vi "IncludeProject.vi"(8 "error in (no error)":errorcluster, 10 "Path":path, 11 "Whitelist in":refnum<class "Whitelist.lvclass">) -> (0 "error out":errorcluster, 3 "Whitelist out":refnum<class "Whitelist.lvclass">)   [LabVIEW 2019, in "Whitelist.lvclass"]
doc: "Includes files from a project in the whitelist."
uses:
  Whitelist.lvclass
  Whitelist.lvclass/Whitelist.ctl
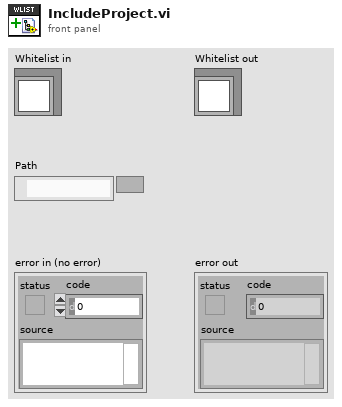
[diagram p1: front panel]
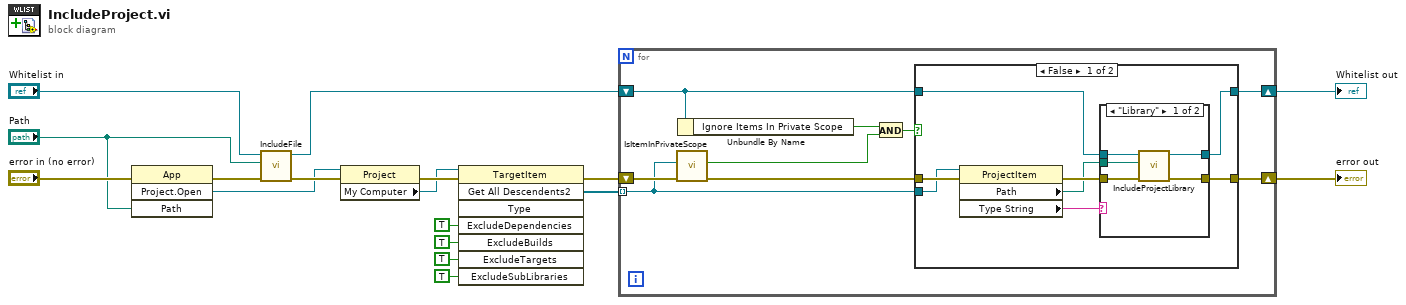
[diagram p0: block diagram]
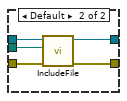
[diagram p2: hidden frame]
diagram:
  n1 = invoke class="App" method="Project.Open"(error in="error in (no error)", "Path"="Path") -> (error out=w16:errorcluster, "Project:Open"=w10:refnum<vi>)  [unwired: 2 in, 2 out]
  n2 = call "IncludeFile.vi"("error in (no error)"=w16, "Path"="Path", "Whitelist in"="Whitelist in") -> ("error out"=w15:errorcluster, "Whitelist out"=w4:refnum<class "Whitelist.lvclass">)  [unwired: 7 in]
  n3 = property class="Project"(reference=w10, error in=w15) -> (error out=w11:errorcluster, "My Computer"=w9:refnum<vi>)  [unwired: 1 out]
  n4 = invoke class="TargetItem" method="Get All Descendents2"(reference=w9, error in=w11, "ExcludeDependencies"=TRUE, "ExcludeBuilds"=TRUE, "ExcludeTargets"=TRUE, "ExcludeSubLibraries"=TRUE) -> (error out=w12:errorcluster, "Get All Descendents2"=w2:refnum<vi>[])  [unwired: 2 in, 6 out]
  n5 = for {
    shift-right: [w26] -> w5
    shift-left: w12 -> [w24]
    shift-right: [w25] -> w3
    shift-left: w4 -> [w20]
    tunnel: w2 -> [w22] mode=indexing
    n6 = call "IsItemInPrivateScope.vi"("error in (no error)"=w24, "Item"=w22) -> ("error out"=w23:errorcluster, "Is Private?"=w19:bool)  [unwired: 8 in]
    n7 = Unbundle By Name(w20) -> ("Ignore Items In Private Scope"=w21:bool)
    n8 = And(x=w21, y=w19) -> (x .and. y?=w18:bool)
    n9 = case shown="False" w18 {
      tunnel: [w34 w45] -> w26
      tunnel: [w33 w46] -> w25
      tunnel: w23 -> [w30 w45]
      tunnel: w22 -> [w29 _]
      tunnel: w20 -> [w28 w46]
      frame False {
        n10 = property class="ProjectItem"(reference=w29, error in=w30) -> (error out=w32:errorcluster, "Path"=w31:path, "Type String"=w27:string)  [unwired: 1 out]
        n11 = case shown="\"Library\"" w27 {
          tunnel: [w38 w44] -> w34
          tunnel: [w35 w43] -> w33
          tunnel: w32 -> [w39 w42]
          tunnel: w31 -> [w36 w41]
          tunnel: w28 -> [w37 w40]
          frame "Library" {
            n12 = call "IncludeProjectLibrary.vi"("error in (no error)"=w39, "Path"=w36, "Whitelist in"=w37) -> ("error out"=w38:errorcluster, "Whitelist out"=w35:refnum<class "Whitelist.lvclass">)  [unwired: 7 in]
          }
          frame Default {
            n13 = call "IncludeFile.vi"("error in (no error)"=w42, "Path"=w41, "Whitelist in"=w40) -> ("error out"=w44:errorcluster, "Whitelist out"=w43:refnum<class "Whitelist.lvclass">)  [unwired: 7 in]
          }
        }
      }
      frame True {
      }
    }
  }
  "error out" <- w5
  "Whitelist out" <- w3
